vi "Decision_Tree.vi"(0 "Numeric":dbl) -> (1 "Case 1":dbl, 2 "Case 2":dbl)   [LabVIEW 2011]
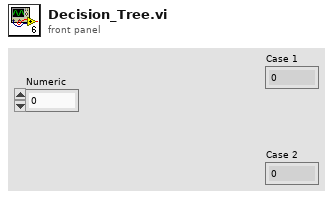
[diagram p1: front panel]
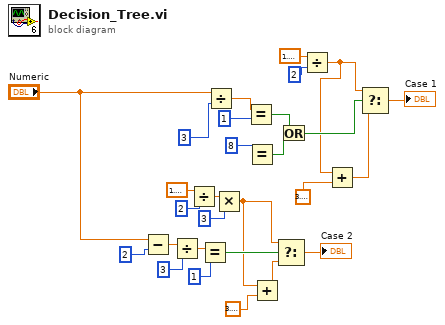
[diagram p0: block diagram]
diagram:
  n1 = Subtract(x="Numeric", y=2) -> (x-y=w15:dbl)
  n2 = Divide(x=w15, y=3) -> (x/y=w13:dbl)
  n3 = Divide(x=1.5707963267948966, y=2) -> (x/y=w6:dbl)
  n4 = Equal?(x=w13, y=1) -> (x = y?=w11:bool)
  n5 = Divide(x="Numeric", y=3) -> (x/y=w26:dbl)
  n6 = Multiply(x=w6, y=3) -> (x*y=w4:dbl)
  n7 = Equal?(x=w26, y=1) -> (x = y?=w24:bool)
  n8 = Equal?(x=8) -> (x = y?=w23:bool)  [unwired: 1 in]
  n9 = Add(x=w4, y=3.141592653589793) -> (x+y=w7:dbl)
  n10 = Select(t=w4, s=w11, f=w7) -> (s? t:f=→"Case 2":dbl)
  n11 = Or(x=w24, y=w23) -> (x .or. y?=w22:bool)
  n12 = Divide(x=1.5707963267948966, y=2) -> (x/y=w18:dbl)
  n13 = Add(x=w18, y=3.141592653589793) -> (x+y=w17:dbl)
  n14 = Select(t=w18, s=w22, f=w17) -> (s? t:f=→"Case 1":dbl)
